vi "bench_ini.vi"(11 "Path":path) -> ()   [LabVIEW 2014]
uses:
  <vilib>/Utility/config.llb/Read Key (String).vi
  GLOBAL_BENCH.vi
  <vilib>/Utility/config.llb/NI_LVConfig.lvlib
panel:
  out "BENCH_PARAMS":T1
  out "num incremental":string
  out "num de serie":string
  out "no banc":string
  out "mois":string
  out "annee":string
  out "date string":string
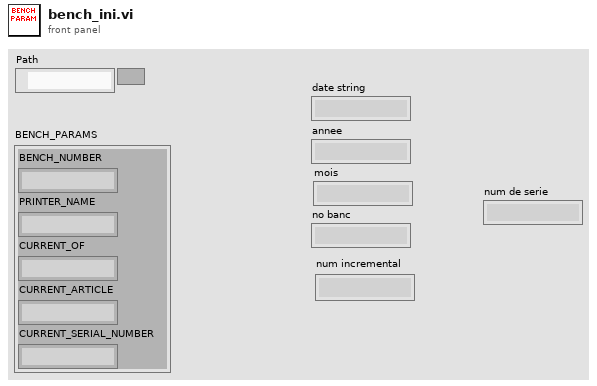
[diagram p1: front panel]
types:
  T1 = cluster{"BENCH_NUMBER":string, "PRINTER_NAME":string, "CURRENT_OF":string, "CURRENT_ARTICLE":string, "CURRENT_SERIAL_NUMBER":string}
  T2 = typedef "NI_LVConfig.lvlib/Config Data RefNum.ctl" = refnum<k1>
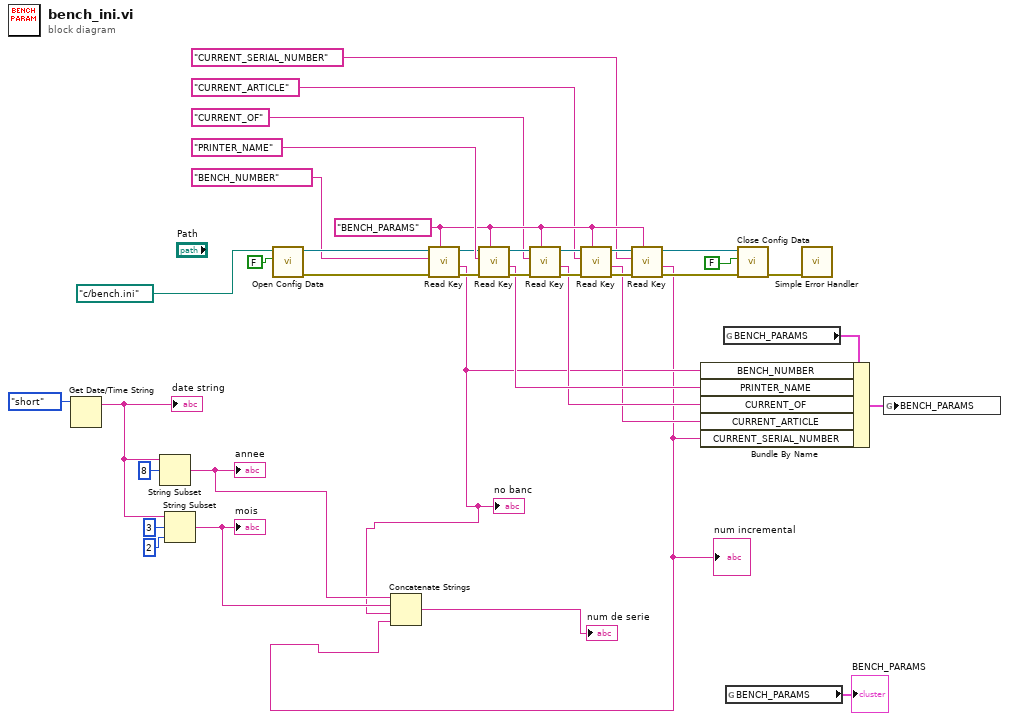
[diagram p0: block diagram]
diagram:
  w21 = "BENCH_PARAMS" ("section")
  n1 = Get Date/Time String(date format (0)=enum16{"short", "long", "abbreviated"}."short") -> (date string=w8:string)  [unwired: 2 in, 1 out]
  "date string" <- w8
  n2 = String Subset(string=w8, offset (0)=8) -> (substring=w6:string)  [unwired: 1 in]
  "annee" <- w6
  n3 = String Subset(string=w8, offset (0)=3, length (rest)=2 ("length (rest)")) -> (substring=w5:string)
  "mois" <- w5
  n4 = call <vilib>:"Open Config Data.vi"("create file if necessary (T)"=FALSE ("create file if necessary? (T)"), "configuration file path"=path "c:/bench.ini") -> ("error out"=w34:errorcluster, "refnum"=w35:T2)  [unwired: 7 in, 1 out]
  n5 = call-poly <vilib>:"Read Key.vi"("section"=w21, "error in (no error)"=w34, "key"="BENCH_NUMBER" ("Key 1"), "refnum"=w35) -> ("error out"=w30:errorcluster, "value"=w4:string, "refnum out"=w31:T2)  [unwired: 4 in, 1 out]
  "no banc" <- w4
  n6 = call-poly <vilib>:"Read Key.vi"("section"=w21, "error in (no error)"=w30, "key"="PRINTER_NAME" ("Key 1"), "refnum"=w31) -> ("error out"=w25:errorcluster, "value"=w15:string, "refnum out"=w29:T2)  [unwired: 4 in, 1 out]
  n7 = call-poly <vilib>:"Read Key.vi"("section"=w21, "error in (no error)"=w25, "key"="CURRENT_OF" ("Key 5"), "refnum"=w29) -> ("error out"=w24:errorcluster, "value"=w14:string, "refnum out"=w28:T2)  [unwired: 4 in, 1 out]
  n8 = call-poly <vilib>:"Read Key.vi"("section"=w21, "error in (no error)"=w24, "key"="CURRENT_ARTICLE" ("Key 2"), "refnum"=w28) -> ("error out"=w23:errorcluster, "value"=w13:string, "refnum out"=w27:T2)  [unwired: 4 in, 1 out]
  n9 = call-poly <vilib>:"Read Key.vi"("section"=w21, "error in (no error)"=w23, "key"="CURRENT_SERIAL_NUMBER" ("Key 3"), "refnum"=w27) -> ("error out"=w22:errorcluster, "value"=w2:string, "refnum out"=w26:T2)  [unwired: 4 in, 1 out]
  "num incremental" <- w2
  n10 = Concatenate Strings(w6, w5, w4, w2) -> (→"num de serie":string)
  n11 = global read "GLOBAL_BENCH.vi" "BENCH_PARAMS"() -> (w16:T1)
  n12 = Bundle By Name(cluster=w16, "BENCH_NUMBER"=w4, "PRINTER_NAME"=w15, "CURRENT_OF"=w14, "CURRENT_ARTICLE"=w13, "CURRENT_SERIAL_NUMBER"=w2) -> (w17:T1)
  n13 = global read "GLOBAL_BENCH.vi" "BENCH_PARAMS"() -> (→"BENCH_PARAMS":T1)
  n14 = call <vilib>:"Close Config Data.vi"("error in (no error)"=w22, "write file if changed (T)"=FALSE ("write configuration file? (T)"), "refnum"=w26) -> ("error out"=w38:errorcluster)  [unwired: 8 out]
  n15 = call <vilib>:"Simple Error Handler.vi"("error in (no error)"=w38) -> ()  [unwired: 1 in, 8 out]
  n16 = global write "GLOBAL_BENCH.vi" "BENCH_PARAMS"(w17) -> ()
